vi "QCP Reader.vi"(10 "Path Relative?":bool=TRUE, 11 "File Path":string="AutoQCP.csv") -> ()   [LabVIEW 2015]
uses:
  <userlib>/836-Library/System/QCP Support Code/QCP_Get_DBL.vi
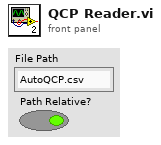
[diagram p1: front panel]
types:
  T1 = typedef "QCP Data Block.ctl" = refnum<data-value>
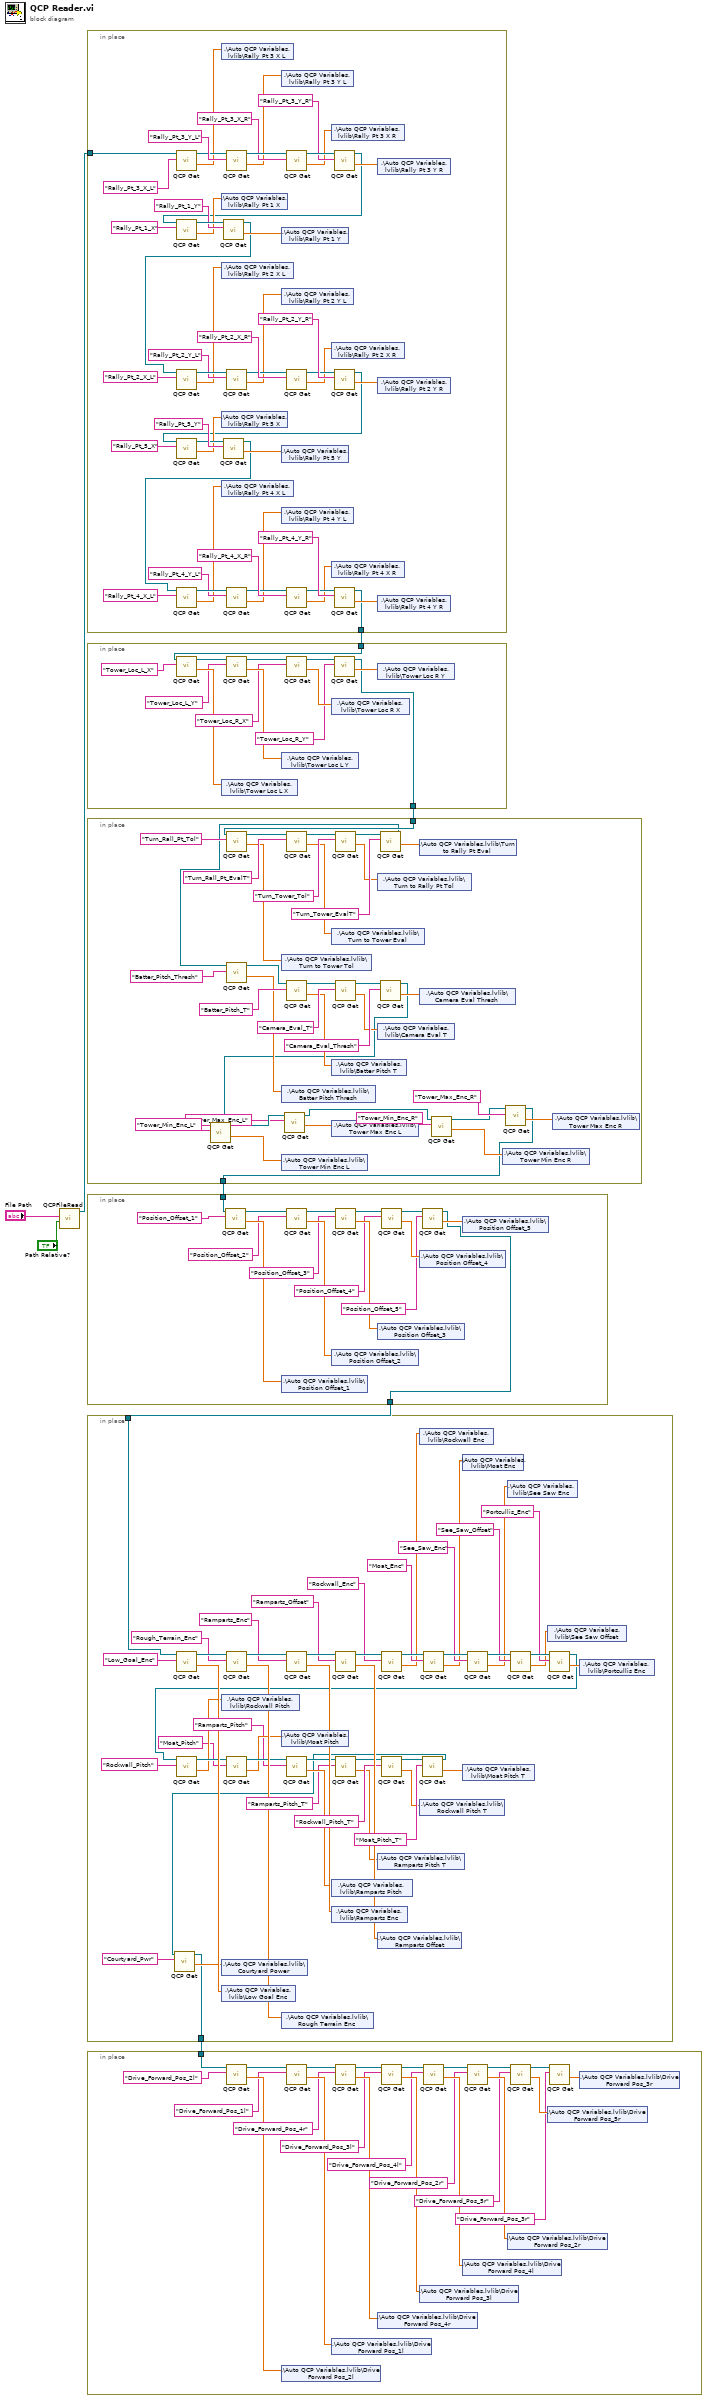
[diagram p0: block diagram]
diagram:
  n1 = call <userlib>:"QCPFileRead.vi"("Path Relative?"="Path Relative?", "File Path"="File Path") -> ("QCP Data Block Out"=w7:T1)  [unwired: 8 in, 1 out]
  n2 = in-place {
    in-place-border: w7 -> [w30]
    in-place-border: [w9] -> w5
    n3 = call-poly <userlib>:"QCP Get.vi"("QCP Data Block In"=w30, "QCP Name"="Rally_Pt_3_X_L") -> ("QCP Data Block Out"=w41:T1, "Value Out"=w22:dbl)  [unwired: 6 in, 1 out]
    n4 = shared-variable ".\\Auto QCP Variables.lvlib\\Rally Pt 3 X L"(w22) -> ()  [unwired: 1 in, 1 out]
    n5 = call-poly <userlib>:"QCP Get.vi"("QCP Data Block In"=w41, "QCP Name"="Rally_Pt_3_Y_L") -> ("QCP Data Block Out"=w47:T1, "Value Out"=w24:dbl)  [unwired: 6 in, 1 out]
    n6 = shared-variable ".\\Auto QCP Variables.lvlib\\Rally Pt 3 Y L"(w24) -> ()  [unwired: 1 in, 1 out]
    n7 = call-poly <userlib>:"QCP Get.vi"("QCP Data Block In"=w47, "QCP Name"="Rally_Pt_3_X_R") -> ("QCP Data Block Out"=w46:T1, "Value Out"=w23:dbl)  [unwired: 6 in, 1 out]
    n8 = shared-variable ".\\Auto QCP Variables.lvlib\\Rally Pt 3 X R"(w23) -> ()  [unwired: 1 in, 1 out]
    n9 = call-poly <userlib>:"QCP Get.vi"("QCP Data Block In"=w46, "QCP Name"="Rally_Pt_3_Y_R") -> ("QCP Data Block Out"=w13:T1, "Value Out"=w25:dbl)  [unwired: 6 in, 1 out]
    n10 = call-poly <userlib>:"QCP Get.vi"("QCP Data Block In"=w13, "QCP Name"="Rally_Pt_1_X") -> ("QCP Data Block Out"=w57:T1, "Value Out"=w29:dbl)  [unwired: 6 in, 1 out]
    n11 = shared-variable ".\\Auto QCP Variables.lvlib\\Rally Pt 1 X"(w29) -> ()  [unwired: 1 in, 1 out]
    n12 = call-poly <userlib>:"QCP Get.vi"("QCP Data Block In"=w57, "QCP Name"="Rally_Pt_1_Y") -> ("QCP Data Block Out"=w12:T1, "Value Out"=w28:dbl)  [unwired: 6 in, 1 out]
    n13 = call-poly <userlib>:"QCP Get.vi"("QCP Data Block In"=w12, "QCP Name"="Rally_Pt_2_X_L") -> ("QCP Data Block Out"=w56:T1, "Value Out"=w14:dbl)  [unwired: 6 in, 1 out]
    n14 = shared-variable ".\\Auto QCP Variables.lvlib\\Rally Pt 2 X L"(w14) -> ()  [unwired: 1 in, 1 out]
    n15 = call-poly <userlib>:"QCP Get.vi"("QCP Data Block In"=w56, "QCP Name"="Rally_Pt_2_Y_L") -> ("QCP Data Block Out"=w48:T1, "Value Out"=w16:dbl)  [unwired: 6 in, 1 out]
    n16 = shared-variable ".\\Auto QCP Variables.lvlib\\Rally Pt 1 Y"(w28) -> ()  [unwired: 1 in, 1 out]
    n17 = shared-variable ".\\Auto QCP Variables.lvlib\\Rally Pt 2 Y L"(w16) -> ()  [unwired: 1 in, 1 out]
    n18 = call-poly <userlib>:"QCP Get.vi"("QCP Data Block In"=w48, "QCP Name"="Rally_Pt_2_X_R") -> ("QCP Data Block Out"=w49:T1, "Value Out"=w15:dbl)  [unwired: 6 in, 1 out]
    n19 = shared-variable ".\\Auto QCP Variables.lvlib\\Rally Pt 2 X R"(w15) -> ()  [unwired: 1 in, 1 out]
    n20 = call-poly <userlib>:"QCP Get.vi"("QCP Data Block In"=w49, "QCP Name"="Rally_Pt_2_Y_R") -> ("QCP Data Block Out"=w11:T1, "Value Out"=w17:dbl)  [unwired: 6 in, 1 out]
    n21 = call-poly <userlib>:"QCP Get.vi"("QCP Data Block In"=w11, "QCP Name"="Rally_Pt_5_X") -> ("QCP Data Block Out"=w31:T1, "Value Out"=w27:dbl)  [unwired: 6 in, 1 out]
    n22 = shared-variable ".\\Auto QCP Variables.lvlib\\Rally Pt 5 X"(w27) -> ()  [unwired: 1 in, 1 out]
    n23 = call-poly <userlib>:"QCP Get.vi"("QCP Data Block In"=w31, "QCP Name"="Rally_Pt_5_Y") -> ("QCP Data Block Out"=w10:T1, "Value Out"=w26:dbl)  [unwired: 6 in, 1 out]
    n24 = call-poly <userlib>:"QCP Get.vi"("QCP Data Block In"=w10, "QCP Name"="Rally_Pt_4_X_L") -> ("QCP Data Block Out"=w40:T1, "Value Out"=w18:dbl)  [unwired: 6 in, 1 out]
    n25 = shared-variable ".\\Auto QCP Variables.lvlib\\Rally Pt 4 X L"(w18) -> ()  [unwired: 1 in, 1 out]
    n26 = call-poly <userlib>:"QCP Get.vi"("QCP Data Block In"=w40, "QCP Name"="Rally_Pt_4_Y_L") -> ("QCP Data Block Out"=w34:T1, "Value Out"=w19:dbl)  [unwired: 6 in, 1 out]
    n27 = shared-variable ".\\Auto QCP Variables.lvlib\\Rally Pt 5 Y"(w26) -> ()  [unwired: 1 in, 1 out]
    n28 = shared-variable ".\\Auto QCP Variables.lvlib\\Rally Pt 4 Y L"(w19) -> ()  [unwired: 1 in, 1 out]
    n29 = call-poly <userlib>:"QCP Get.vi"("QCP Data Block In"=w34, "QCP Name"="Rally_Pt_4_X_R") -> ("QCP Data Block Out"=w35:T1, "Value Out"=w21:dbl)  [unwired: 6 in, 1 out]
    n30 = shared-variable ".\\Auto QCP Variables.lvlib\\Rally Pt 4 X R"(w21) -> ()  [unwired: 1 in, 1 out]
    n31 = call-poly <userlib>:"QCP Get.vi"("QCP Data Block In"=w35, "QCP Name"="Rally_Pt_4_Y_R") -> ("QCP Data Block Out"=w9:T1, "Value Out"=w20:dbl)  [unwired: 6 in, 1 out]
    n32 = shared-variable ".\\Auto QCP Variables.lvlib\\Rally Pt 3 Y R"(w25) -> ()  [unwired: 1 in, 1 out]
    n33 = shared-variable ".\\Auto QCP Variables.lvlib\\Rally Pt 2 Y R"(w17) -> ()  [unwired: 1 in, 1 out]
    n34 = shared-variable ".\\Auto QCP Variables.lvlib\\Rally Pt 4 Y R"(w20) -> ()  [unwired: 1 in, 1 out]
  }
  n35 = in-place {
    in-place-border: w5 -> [w59]
    in-place-border: [w58] -> w4
    n36 = call-poly <userlib>:"QCP Get.vi"("QCP Data Block In"=w59, "QCP Name"="Tower_Loc_L_X") -> ("QCP Data Block Out"=w69:T1, "Value Out"=w64:dbl)  [unwired: 6 in, 1 out]
    n37 = shared-variable ".\\Auto QCP Variables.lvlib\\Tower Loc L X"(w64) -> ()  [unwired: 1 in, 1 out]
    n38 = call-poly <userlib>:"QCP Get.vi"("QCP Data Block In"=w69, "QCP Name"="Tower_Loc_L_Y") -> ("QCP Data Block Out"=w68:T1, "Value Out"=w65:dbl)  [unwired: 6 in, 1 out]
    n39 = shared-variable ".\\Auto QCP Variables.lvlib\\Tower Loc L Y"(w65) -> ()  [unwired: 1 in, 1 out]
    n40 = call-poly <userlib>:"QCP Get.vi"("QCP Data Block In"=w68, "QCP Name"="Tower_Loc_R_X") -> ("QCP Data Block Out"=w70:T1, "Value Out"=w66:dbl)  [unwired: 6 in, 1 out]
    n41 = shared-variable ".\\Auto QCP Variables.lvlib\\Tower Loc R X"(w66) -> ()  [unwired: 1 in, 1 out]
    n42 = call-poly <userlib>:"QCP Get.vi"("QCP Data Block In"=w70, "QCP Name"="Tower_Loc_R_Y") -> ("QCP Data Block Out"=w58:T1, "Value Out"=w67:dbl)  [unwired: 6 in, 1 out]
    n43 = shared-variable ".\\Auto QCP Variables.lvlib\\Tower Loc R Y"(w67) -> ()  [unwired: 1 in, 1 out]
  }
  n44 = in-place {
    in-place-border: w4 -> [w80]
    in-place-border: [w71] -> w3
    n45 = call-poly <userlib>:"QCP Get.vi"("QCP Data Block In"=w80, "QCP Name"="Turn_Rall_Pt_Tol") -> ("QCP Data Block Out"=w106:T1, "Value Out"=w93:dbl)  [unwired: 6 in, 1 out]
    n46 = shared-variable ".\\Auto QCP Variables.lvlib\\Turn to Tower Tol"(w93) -> ()  [unwired: 1 in, 1 out]
    n47 = call-poly <userlib>:"QCP Get.vi"("QCP Data Block In"=w106, "QCP Name"="Turn_Rall_Pt_EvalT") -> ("QCP Data Block Out"=w101:T1, "Value Out"=w92:dbl)  [unwired: 6 in, 1 out]
    n48 = shared-variable ".\\Auto QCP Variables.lvlib\\Turn to Tower Eval"(w92) -> ()  [unwired: 1 in, 1 out]
    n49 = call-poly <userlib>:"QCP Get.vi"("QCP Data Block In"=w101, "QCP Name"="Turn_Tower_Tol") -> ("QCP Data Block Out"=w103:T1, "Value Out"=w91:dbl)  [unwired: 6 in, 1 out]
    n50 = shared-variable ".\\Auto QCP Variables.lvlib\\Turn to Rally Pt Tol"(w91) -> ()  [unwired: 1 in, 1 out]
    n51 = call-poly <userlib>:"QCP Get.vi"("QCP Data Block In"=w103, "QCP Name"="Turn_Tower_EvalT") -> ("QCP Data Block Out"=w79:T1, "Value Out"=w90:dbl)  [unwired: 6 in, 1 out]
    n52 = call-poly <userlib>:"QCP Get.vi"("QCP Data Block In"=w79, "QCP Name"="Batter_Pitch_Thresh") -> ("QCP Data Block Out"=w89:T1, "Value Out"=w85:dbl)  [unwired: 6 in, 1 out]
    n53 = shared-variable ".\\Auto QCP Variables.lvlib\\Batter Pitch Thresh"(w85) -> ()  [unwired: 1 in, 1 out]
    n54 = call-poly <userlib>:"QCP Get.vi"("QCP Data Block In"=w89, "QCP Name"="Batter_Pitch_T") -> ("QCP Data Block Out"=w88:T1, "Value Out"=w86:dbl)  [unwired: 6 in, 1 out]
    n55 = shared-variable ".\\Auto QCP Variables.lvlib\\Batter Pitch T"(w86) -> ()  [unwired: 1 in, 1 out]
    n56 = call-poly <userlib>:"QCP Get.vi"("QCP Data Block In"=w88, "QCP Name"="Camera_Eval_T") -> ("QCP Data Block Out"=w98:T1, "Value Out"=w83:dbl)  [unwired: 6 in, 1 out]
    n57 = shared-variable ".\\Auto QCP Variables.lvlib\\Camera Eval T"(w83) -> ()  [unwired: 1 in, 1 out]
    n58 = call-poly <userlib>:"QCP Get.vi"("QCP Data Block In"=w98, "QCP Name"="Camera_Eval_Thresh") -> ("QCP Data Block Out"=w78:T1, "Value Out"=w84:dbl)  [unwired: 6 in, 1 out]
    n59 = call-poly <userlib>:"QCP Get.vi"("QCP Data Block In"=w78, "QCP Name"="Tower_Min_Enc_L") -> ("QCP Data Block Out"=w96:T1, "Value Out"=w81:dbl)  [unwired: 6 in, 1 out]
    n60 = shared-variable ".\\Auto QCP Variables.lvlib\\Tower Min Enc L"(w81) -> ()  [unwired: 1 in, 1 out]
    n61 = call-poly <userlib>:"QCP Get.vi"("QCP Data Block In"=w96, "QCP Name"="Tower_Max_Enc_L") -> ("QCP Data Block Out"=w72:T1, "Value Out"=w82:dbl)  [unwired: 6 in, 1 out]
    n62 = shared-variable ".\\Auto QCP Variables.lvlib\\Tower Max Enc L"(w82) -> ()  [unwired: 1 in, 1 out]
    n63 = shared-variable ".\\Auto QCP Variables.lvlib\\Turn to Rally Pt Eval"(w90) -> ()  [unwired: 1 in, 1 out]
    n64 = shared-variable ".\\Auto QCP Variables.lvlib\\Camera Eval Thresh"(w84) -> ()  [unwired: 1 in, 1 out]
    n65 = call-poly <userlib>:"QCP Get.vi"("QCP Data Block In"=w72, "QCP Name"="Tower_Min_Enc_R") -> ("QCP Data Block Out"=w73:T1, "Value Out"=w77:dbl)  [unwired: 6 in, 1 out]
    n66 = shared-variable ".\\Auto QCP Variables.lvlib\\Tower Min Enc R"(w77) -> ()  [unwired: 1 in, 1 out]
    n67 = call-poly <userlib>:"QCP Get.vi"("QCP Data Block In"=w73, "QCP Name"="Tower_Max_Enc_R") -> ("QCP Data Block Out"=w71:T1, "Value Out"=w76:dbl)  [unwired: 6 in, 1 out]
    n68 = shared-variable ".\\Auto QCP Variables.lvlib\\Tower Max Enc R"(w76) -> ()  [unwired: 1 in, 1 out]
  }
  n69 = in-place {
    in-place-border: w3 -> [w109]
    in-place-border: [w108] -> w2
    n70 = call-poly <userlib>:"QCP Get.vi"("QCP Data Block In"=w109, "QCP Name"="Position_Offset_1") -> ("QCP Data Block Out"=w122:T1, "Value Out"=w123:dbl)  [unwired: 6 in, 1 out]
    n71 = shared-variable ".\\Auto QCP Variables.lvlib\\Position Offset_1"(w123) -> ()  [unwired: 1 in, 1 out]
    n72 = call-poly <userlib>:"QCP Get.vi"("QCP Data Block In"=w122, "QCP Name"="Position_Offset_2") -> ("QCP Data Block Out"=w121:T1, "Value Out"=w118:dbl)  [unwired: 6 in, 1 out]
    n73 = shared-variable ".\\Auto QCP Variables.lvlib\\Position Offset_2"(w118) -> ()  [unwired: 1 in, 1 out]
    n74 = call-poly <userlib>:"QCP Get.vi"("QCP Data Block In"=w121, "QCP Name"="Position_Offset_3") -> ("QCP Data Block Out"=w120:T1, "Value Out"=w117:dbl)  [unwired: 6 in, 1 out]
    n75 = shared-variable ".\\Auto QCP Variables.lvlib\\Position Offset_3"(w117) -> ()  [unwired: 1 in, 1 out]
    n76 = call-poly <userlib>:"QCP Get.vi"("QCP Data Block In"=w120, "QCP Name"="Position_Offset_4") -> ("QCP Data Block Out"=w119:T1, "Value Out"=w116:dbl)  [unwired: 6 in, 1 out]
    n77 = shared-variable ".\\Auto QCP Variables.lvlib\\Position Offset_4"(w116) -> ()  [unwired: 1 in, 1 out]
    n78 = call-poly <userlib>:"QCP Get.vi"("QCP Data Block In"=w119, "QCP Name"="Position_Offset_5") -> ("QCP Data Block Out"=w108:T1, "Value Out"=w115:dbl)  [unwired: 6 in, 1 out]
    n79 = shared-variable ".\\Auto QCP Variables.lvlib\\Position Offset_5"(w115) -> ()  [unwired: 1 in, 1 out]
  }
  n80 = in-place {
    in-place-border: w2 -> [w127]
    in-place-border: [w124] -> w1
    n81 = call-poly <userlib>:"QCP Get.vi"("QCP Data Block In"=w127, "QCP Name"="Low_Goal_Enc") -> ("QCP Data Block Out"=w172:T1, "Value Out"=w147:dbl)  [unwired: 6 in, 1 out]
    n82 = shared-variable ".\\Auto QCP Variables.lvlib\\Low Goal Enc"(w147) -> ()  [unwired: 1 in, 1 out]
    n83 = call-poly <userlib>:"QCP Get.vi"("QCP Data Block In"=w172, "QCP Name"="Rough_Terrain_Enc") -> ("QCP Data Block Out"=w171:T1, "Value Out"=w152:dbl)  [unwired: 6 in, 1 out]
    n84 = shared-variable ".\\Auto QCP Variables.lvlib\\Rough Terrain Enc"(w152) -> ()  [unwired: 1 in, 1 out]
    n85 = call-poly <userlib>:"QCP Get.vi"("QCP Data Block In"=w171, "QCP Name"="Ramparts_Enc") -> ("QCP Data Block Out"=w168:T1, "Value Out"=w150:dbl)  [unwired: 6 in, 1 out]
    n86 = shared-variable ".\\Auto QCP Variables.lvlib\\Ramparts Enc"(w150) -> ()  [unwired: 1 in, 1 out]
    n87 = call-poly <userlib>:"QCP Get.vi"("QCP Data Block In"=w168, "QCP Name"="Ramparts_Offset") -> ("QCP Data Block Out"=w169:T1, "Value Out"=w145:dbl)  [unwired: 6 in, 1 out]
    n88 = shared-variable ".\\Auto QCP Variables.lvlib\\Ramparts Offset"(w145) -> ()  [unwired: 1 in, 1 out]
    n89 = call-poly <userlib>:"QCP Get.vi"("QCP Data Block In"=w169, "QCP Name"="Rockwall_Enc") -> ("QCP Data Block Out"=w170:T1, "Value Out"=w151:dbl)  [unwired: 6 in, 1 out]
    n90 = shared-variable ".\\Auto QCP Variables.lvlib\\Rockwall Enc"(w151) -> ()  [unwired: 1 in, 1 out]
    n91 = call-poly <userlib>:"QCP Get.vi"("QCP Data Block In"=w170, "QCP Name"="Moat_Enc") -> ("QCP Data Block Out"=w165:T1, "Value Out"=w148:dbl)  [unwired: 6 in, 1 out]
    n92 = shared-variable ".\\Auto QCP Variables.lvlib\\Moat Enc"(w148) -> ()  [unwired: 1 in, 1 out]
    n93 = call-poly <userlib>:"QCP Get.vi"("QCP Data Block In"=w165, "QCP Name"="See_Saw_Enc") -> ("QCP Data Block Out"=w167:T1, "Value Out"=w153:dbl)  [unwired: 6 in, 1 out]
    n94 = shared-variable ".\\Auto QCP Variables.lvlib\\See Saw Enc"(w153) -> ()  [unwired: 1 in, 1 out]
    n95 = call-poly <userlib>:"QCP Get.vi"("QCP Data Block In"=w167, "QCP Name"="See_Saw_Offset") -> ("QCP Data Block Out"=w166:T1, "Value Out"=w154:dbl)  [unwired: 6 in, 1 out]
    n96 = shared-variable ".\\Auto QCP Variables.lvlib\\See Saw Offset"(w154) -> ()  [unwired: 1 in, 1 out]
    n97 = call-poly <userlib>:"QCP Get.vi"("QCP Data Block In"=w166, "QCP Name"="Portcullis_Enc") -> ("QCP Data Block Out"=w126:T1, "Value Out"=w149:dbl)  [unwired: 6 in, 1 out]
    n98 = call-poly <userlib>:"QCP Get.vi"("QCP Data Block In"=w126, "QCP Name"="Rockwall_Pitch") -> ("QCP Data Block Out"=w144:T1, "Value Out"=w141:dbl)  [unwired: 6 in, 1 out]
    n99 = shared-variable ".\\Auto QCP Variables.lvlib\\Rockwall Pitch"(w141) -> ()  [unwired: 1 in, 1 out]
    n100 = call-poly <userlib>:"QCP Get.vi"("QCP Data Block In"=w144, "QCP Name"="Moat_Pitch") -> ("QCP Data Block Out"=w143:T1, "Value Out"=w139:dbl)  [unwired: 6 in, 1 out]
    n101 = shared-variable ".\\Auto QCP Variables.lvlib\\Moat Pitch"(w139) -> ()  [unwired: 1 in, 1 out]
    n102 = call-poly <userlib>:"QCP Get.vi"("QCP Data Block In"=w143, "QCP Name"="Ramparts_Pitch") -> ("QCP Data Block Out"=w136:T1, "Value Out"=w137:dbl)  [unwired: 6 in, 1 out]
    n103 = shared-variable ".\\Auto QCP Variables.lvlib\\Ramparts Pitch"(w137) -> ()  [unwired: 1 in, 1 out]
    n104 = call-poly <userlib>:"QCP Get.vi"("QCP Data Block In"=w136, "QCP Name"="Ramparts_Pitch_T") -> ("QCP Data Block Out"=w135:T1, "Value Out"=w129:dbl)  [unwired: 6 in, 1 out]
    n105 = shared-variable ".\\Auto QCP Variables.lvlib\\Ramparts Pitch T"(w129) -> ()  [unwired: 1 in, 1 out]
    n106 = call-poly <userlib>:"QCP Get.vi"("QCP Data Block In"=w135, "QCP Name"="Rockwall_Pitch_T") -> ("QCP Data Block Out"=w134:T1, "Value Out"=w130:dbl)  [unwired: 6 in, 1 out]
    n107 = shared-variable ".\\Auto QCP Variables.lvlib\\Rockwall Pitch T"(w130) -> ()  [unwired: 1 in, 1 out]
    n108 = call-poly <userlib>:"QCP Get.vi"("QCP Data Block In"=w134, "QCP Name"="Moat_Pitch_T") -> ("QCP Data Block Out"=w125:T1, "Value Out"=w128:dbl)  [unwired: 6 in, 1 out]
    n109 = call-poly <userlib>:"QCP Get.vi"("QCP Data Block In"=w125, "QCP Name"="Courtyard_Pwr") -> ("QCP Data Block Out"=w124:T1, "Value Out"=w146:dbl)  [unwired: 6 in, 1 out]
    n110 = shared-variable ".\\Auto QCP Variables.lvlib\\Courtyard Power"(w146) -> ()  [unwired: 1 in, 1 out]
    n111 = shared-variable ".\\Auto QCP Variables.lvlib\\Moat Pitch T"(w128) -> ()  [unwired: 1 in, 1 out]
    n112 = shared-variable ".\\Auto QCP Variables.lvlib\\Portcullis Enc"(w149) -> ()  [unwired: 1 in, 1 out]
  }
  n113 = in-place {
    in-place-border: w1 -> [w173]
    n114 = call-poly <userlib>:"QCP Get.vi"("QCP Data Block In"=w173, "QCP Name"="Drive_Forward_Pos_2l") -> ("QCP Data Block Out"=w196:T1, "Value Out"=w189:dbl)  [unwired: 6 in, 1 out]
    n115 = shared-variable ".\\Auto QCP Variables.lvlib\\Drive Forward Pos_2l"(w189) -> ()  [unwired: 1 in, 1 out]
    n116 = call-poly <userlib>:"QCP Get.vi"("QCP Data Block In"=w196, "QCP Name"="Drive_Forward_Pos_1l") -> ("QCP Data Block Out"=w195:T1, "Value Out"=w188:dbl)  [unwired: 6 in, 1 out]
    n117 = shared-variable ".\\Auto QCP Variables.lvlib\\Drive Forward Pos_1l"(w188) -> ()  [unwired: 1 in, 1 out]
    n118 = call-poly <userlib>:"QCP Get.vi"("QCP Data Block In"=w195, "QCP Name"="Drive_Forward_Pos_4r") -> ("QCP Data Block Out"=w194:T1, "Value Out"=w187:dbl)  [unwired: 6 in, 1 out]
    n119 = shared-variable ".\\Auto QCP Variables.lvlib\\Drive Forward Pos_4r"(w187) -> ()  [unwired: 1 in, 1 out]
    n120 = call-poly <userlib>:"QCP Get.vi"("QCP Data Block In"=w194, "QCP Name"="Drive_Forward_Pos_3l") -> ("QCP Data Block Out"=w193:T1, "Value Out"=w186:dbl)  [unwired: 6 in, 1 out]
    n121 = shared-variable ".\\Auto QCP Variables.lvlib\\Drive Forward Pos_3l"(w186) -> ()  [unwired: 1 in, 1 out]
    n122 = call-poly <userlib>:"QCP Get.vi"("QCP Data Block In"=w193, "QCP Name"="Drive_Forward_Pos_4l") -> ("QCP Data Block Out"=w192:T1, "Value Out"=w185:dbl)  [unwired: 6 in, 1 out]
    n123 = shared-variable ".\\Auto QCP Variables.lvlib\\Drive Forward Pos_4l"(w185) -> ()  [unwired: 1 in, 1 out]
    n124 = call-poly <userlib>:"QCP Get.vi"("QCP Data Block In"=w192, "QCP Name"="Drive_Forward_Pos_2r") -> ("QCP Data Block Out"=w191:T1, "Value Out"=w184:dbl)  [unwired: 6 in, 1 out]
    n125 = shared-variable ".\\Auto QCP Variables.lvlib\\Drive Forward Pos_2r"(w184) -> ()  [unwired: 1 in, 1 out]
    n126 = call-poly <userlib>:"QCP Get.vi"("QCP Data Block In"=w191, "QCP Name"="Drive_Forward_Pos_5r") -> ("QCP Data Block Out"=w190:T1, "Value Out"=w183:dbl)  [unwired: 6 in, 1 out]
    n127 = shared-variable ".\\Auto QCP Variables.lvlib\\Drive Forward Pos_5r"(w183) -> ()  [unwired: 1 in, 1 out]
    n128 = call-poly <userlib>:"QCP Get.vi"("QCP Data Block In"=w190, "QCP Name"="Drive_Forward_Pos_3r") -> ("Value Out"=w182:dbl)  [unwired: 6 in, 2 out]
    n129 = shared-variable ".\\Auto QCP Variables.lvlib\\Drive Forward Pos_3r"(w182) -> ()  [unwired: 1 in, 1 out]
  }
